vi "cRIO_EPTx_FPGA_MulInj_SCAN.vi"() -> ()   [LabVIEW 2023]
uses:
  C:/Program Files (x86)/National Instruments/LabVIEW 2023/vi.lib/Powertrain Controls/Device Drivers/Engine Position Tracking/EPTx/RevA/FPGA/Controls/EPTxDebug.ctl
  C:/Program Files (x86)/National Instruments/LabVIEW 2023/vi.lib/Powertrain Controls/Device Drivers/Engine Position Tracking/EPTx/RevA/FPGA/Controls/EPTxTooth.ctl
  <vilib>/Powertrain Controls/Device Drivers/Engine Position Tracking/EPTx/RevA/FPGA/Controls/EPTxSignals.ctl
  <vilib>/Powertrain Controls/Device Drivers/Engine Position Tracking/EPTx/RevA/FPGA/Controls/EPTxSupervisor.ctl
  <vilib>/Platform/TimedLoop/XDataNode/timing_clust.ctl
  <vilib>/Platform/TimedLoop/XDataNode/nitl_modes.ctl
  <vilib>/Platform/TimedLoop/XDataNode/wakeup.ctl
  <vilib>/Powertrain Controls/Device Drivers/Engine Position Tracking/EPTx/RevA/FPGA/Controls/EPTxAAPControl.ctl
  <vilib>/Powertrain Controls/Device Drivers/Engine Position Tracking/EPTx/RevA/FPGA/Controls/EPTxPatternConfig.ctl
  <vilib>/Powertrain Controls/Device Drivers/Engine Position Tracking/EPTx/RevA/FPGA/Controls/Patterns.ctl
  <vilib>/Powertrain Controls/Device Drivers/Engine Position Tracking/EPTx/RevA/FPGA/Controls/EPTxControl.ctl
  <vilib>/rvi/Emulation/niFpgaSctlEmulationGetInTimedLoop.vi
  <vilib>/rvi/Emulation/niFpgaEmulationReportErrorSimple.vi
  <vilib>/rvi/Emulation/niFpgaGetClockAttributes.vi
  <vilib>/rvi/Emulation/niFpgaCriticalErrorInLSC.vi
  <vilib>/rvi/eio/common/nirviEmuTemplateMethod_errors.vi
  <vilib>/Platform/TimedLoop/XDataNode/XDataNode.xnode
  <vilib>/eio/EIONode/EIONode.xnode
  <vilib>/Powertrain Controls/Device Drivers/Engine Position Tracking/EPTx/RevA/FPGA/Extras/Command Sequence - 12e.vi
  <vilib>/Platform/TimedLoop/XDataNode/XDNodeRunTimeDep.lvlib
  <vilib>/Powertrain Controls/Device Drivers/Engine Position Tracking/EPTx/RevA/FPGA/EPTx - RevA - FPGA.lvlib
panel:
  out "EPTxSupervisor_FPGA":T1
  out "EPTxSignals":T2
  out "EPTxTooth":T3
  out "EPTxDebug":T4
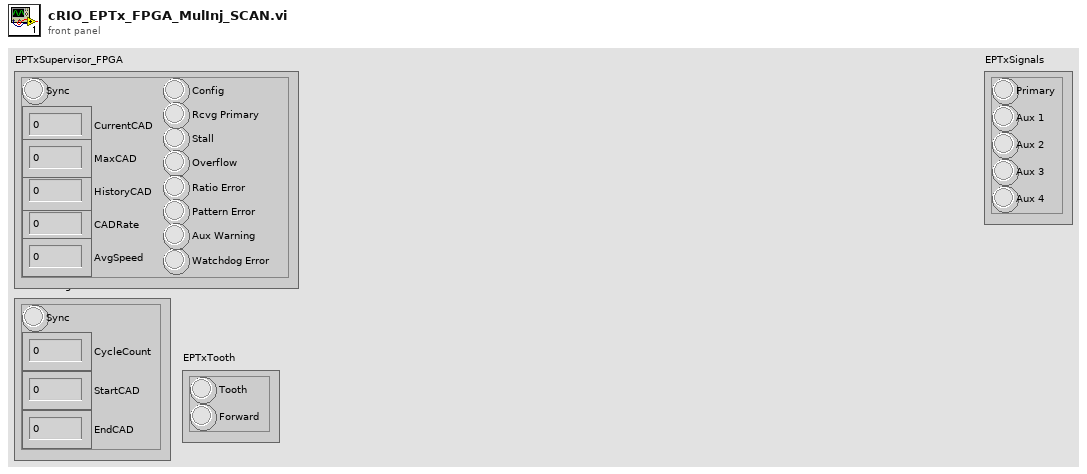
[diagram p1: front panel]
types:
  T1 = typedef "EPTx - RevA - FPGA.lvlib/EPTxSupervisor.ctl" = cluster{"Sync":bool, "CurrentCAD":fxp<+,18,11>, "MaxCAD":fxp<+,11,11>, "HistoryCAD":fxp<+,11,11>, "CADRate":fxp<+,22,8>, "AvgSpeed":fxp<+,17,15>, "Config":bool, "Rcvg Primary":bool, "Stall":bool, "Overflow":bool, "Ratio Error":bool, "Pattern Error":bool, "Aux Warning":bool, "Watchdog Error":bool}
  T2 = typedef "EPTx - RevA - FPGA.lvlib/EPTxSignals.ctl" = cluster{"Primary":bool, "Aux 1":bool, "Aux 2":bool, "Aux 3":bool, "Aux 4":bool}
  T3 = typedef "EPTxTooth.ctl" = cluster{"Tooth":bool, "Forward":bool}
  T4 = typedef "EPTx - RevA - FPGA.lvlib/EPTxDebug.ctl" = cluster{"Sync":bool, "CycleCount":fxp<+,8,8>, "StartCAD":fxp<+,18,11>, "EndCAD":fxp<+,18,11>}
  T5 = typedef "XDNodeRunTimeDep.lvlib/timing_clust.ctl" = cluster{"Expected End [f-1]":u64, "Actual End [f-1]":u64, "Finished Late? [f-1]":bool, "Expected End [i-1]":u64, "Actual End [i-1]":u64, "Finished Late? [i-1]":bool, "Expected Start [i]":u64, "Actual Start [i]":u64, "Expected Start [f]":u64, "Actual Start [f]":u64, "Source Name":string, "Structure Name":string, "Period":i64, "Deadline":i64, "Offset":i64, "Start":i64, "Priority":i32, "Timeout":i32, "Mode":T6, "Wakeup Reason":T7, "Error":errorcluster, "Source Type":string, "Secondary Source Type":string, "Global End Time":u64, "Global Start Time":u64, "Frame Duration":u64, "Iteration Duration":u64, "Assigned CPU":i32, "I/O Scan Engine Mode":u32}
  T6 = typedef "XDNodeRunTimeDep.lvlib/nitl_modes.ctl" = enum32{"No Change", "Process missed periods, maintain original phase", "Discard missed periods, maintain original phase", "Process missed periods, ignore original phase", "Discard missed periods, ignore original phase"}
  T7 = typedef "XDNodeRunTimeDep.lvlib/wakeup.ctl" = enum32{"Normal", "Aborted", "Asynchronous wakeup", "Timing source error", "Timed loop error", "Timeout"}
  T8 = typedef "EPTx - RevA - FPGA.lvlib/EPTxAAPControl.ctl" = cluster{"Enable":bool, "RisingCAD":fxp<+,18,11>, "FallingCAD":fxp<+,18,11>}
  T9 = typedef "EPTx - RevA - FPGA.lvlib/EPTxControl.ctl" = cluster{"Sync Enable":bool, "Clear Errors":bool, "Sim Enable":bool, "Sim Rate":fxp<+,24,6>, "Watchdog":bool}
  T10 = typedef "EPTx - RevA - FPGA.lvlib/Patterns.ctl" = cluster{"Primary":fxp<+,19,12>, "Primary State":bool, "Aux 1":fxp<+,19,12>, "Aux 1 State":bool, "Aux 2":fxp<+,19,12>, "Aux 2 State":bool, "Aux 3":fxp<+,19,12>, "Aux 3 State":bool, "Aux 4":fxp<+,19,12>, "Aux 4 State":bool}
  T11 = typedef "EPTx - RevA - FPGA.lvlib/EPTxPatternConfig.ctl" = cluster{"Address":fxp<+,14,14>, "Pattern":T10}
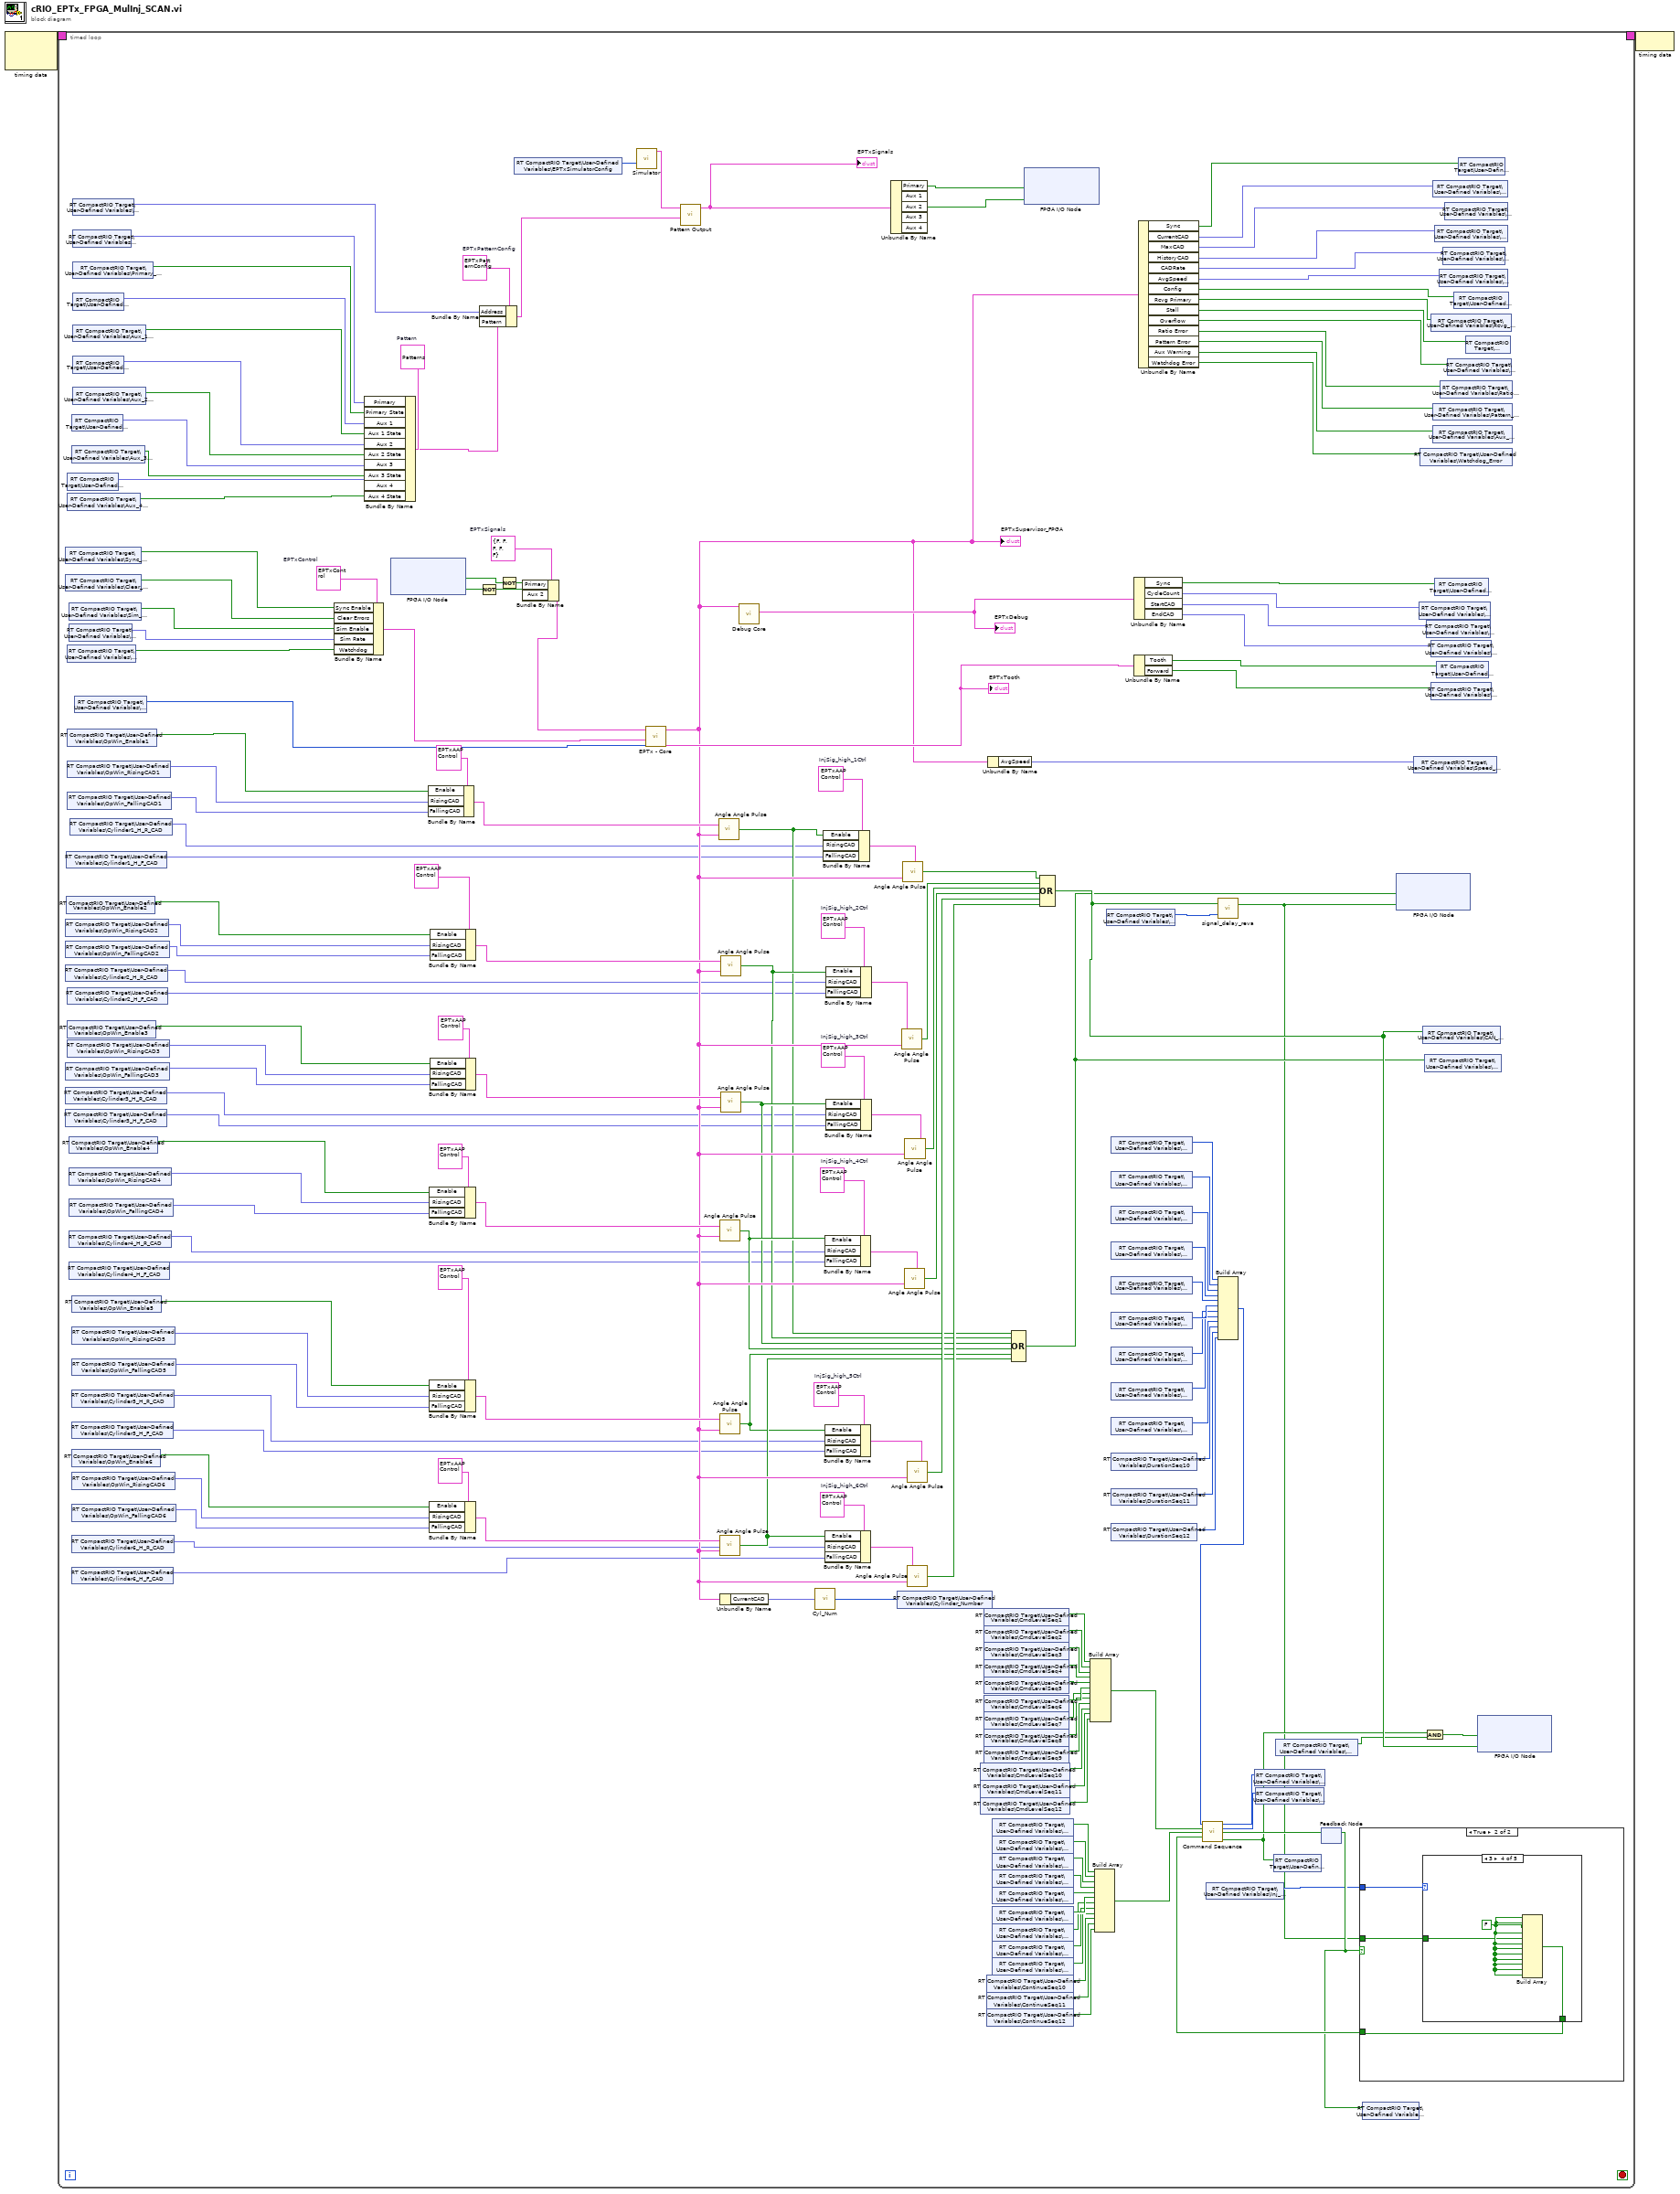
[diagram p0: block diagram]
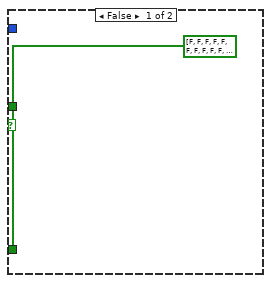
[diagram p2: hidden frame]
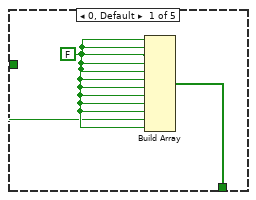
[diagram p3: hidden frame]
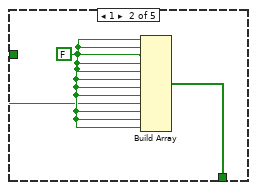
[diagram p4: hidden frame]
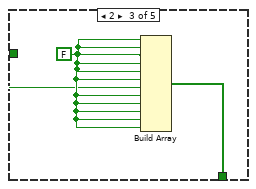
[diagram p5: hidden frame]
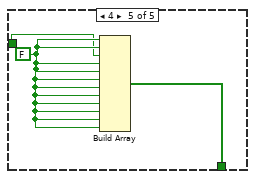
[diagram p6: hidden frame]
diagram:
  n1 = node-c288() -> (w2:T5)  [unwired: 2 in]
  n2 = timed-loop {
    timing: w2 -> [_]
    timing-out: [_] -> w1
    stop <- _ stop-if-true
    w139 = T2 {"Primary"=FALSE, "Aux 1"=FALSE, "Aux 2"=FALSE, "Aux 3"=FALSE, "Aux 4"=FALSE}  # EPTxSignals
    w145 = T8 {"Enable"=FALSE, "RisingCAD"=0.0, "FallingCAD"=0.0}  # InjSig_high_6Ctrl
    w150 = T8 {"Enable"=FALSE, "RisingCAD"=0.0, "FallingCAD"=0.0}  # InjSig_high_5Ctrl
    w153 = T8 {"Enable"=FALSE, "RisingCAD"=0.0, "FallingCAD"=0.0}  # InjSig_high_4Ctrl
    w160 = T8 {"Enable"=FALSE, "RisingCAD"=0.0, "FallingCAD"=0.0}  # InjSig_high_3Ctrl
    w164 = T8 {"Enable"=FALSE, "RisingCAD"=0.0, "FallingCAD"=0.0}  # InjSig_high_2Ctrl
    w168 = T9 {"Sync Enable"=FALSE, "Clear Errors"=FALSE, "Sim Enable"=FALSE, "Sim Rate"=0.0, "Watchdog"=FALSE}  # EPTxControl
    w173 = T10 {"Primary"=0.0, "Primary State"=FALSE, "Aux 1"=0.0, "Aux 1 State"=FALSE, "Aux 2"=0.0, "Aux 2 State"=FALSE, "Aux 3"=0.0, "Aux 3 State"=FALSE, "Aux 4"=0.0, "Aux 4 State"=FALSE}  # Pattern
    w174 = T11 {"Address"=0.0, "Pattern"={"Primary"=0.0, "Primary State"=FALSE, "Aux 1"=0.0, "Aux 1 State"=FALSE, "Aux 2"=0.0, "Aux 2 State"=FALSE, "Aux 3"=0.0, "Aux 3 State"=FALSE, "Aux 4"=0.0, "Aux 4 State"=FALSE}}  # EPTxPatternConfig
    w177 = T8 {"Enable"=FALSE, "RisingCAD"=0.0, "FallingCAD"=0.0}  # InjSig_high_1Ctrl
    n3 = shared-variable "RT CompactRIO Target\\User-Defined Variables\\OpWin_FallingCAD2"() -> (w103:fxp<+/-,32,16>)  [unwired: 1 in, 1 out]
    n4 = shared-variable "RT CompactRIO Target\\User-Defined Variables\\Cylinder3_H_R_CAD"() -> (w97:fxp<+/-,32,16>)  [unwired: 1 in, 1 out]
    n5 = shared-variable "RT CompactRIO Target\\User-Defined Variables\\Sync_Enable"() -> (w116:bool)  [unwired: 1 in, 1 out]
    n6 = shared-variable "RT CompactRIO Target\\User-Defined Variables\\Clear_Errors"() -> (w115:bool)  [unwired: 1 in, 1 out]
    n7 = shared-variable "RT CompactRIO Target\\User-Defined Variables\\OpWin_RisingCAD2"() -> (w104:fxp<+/-,32,16>)  [unwired: 1 in, 1 out]
    n8 = shared-variable "RT CompactRIO Target\\User-Defined Variables\\Cylinder2_H_R_CAD"() -> (w102:fxp<+/-,32,16>)  [unwired: 1 in, 1 out]
    n9 = shared-variable "RT CompactRIO Target\\User-Defined Variables\\OpWin_FallingCAD3"() -> (w98:fxp<+/-,32,16>)  [unwired: 1 in, 1 out]
    n10 = shared-variable "RT CompactRIO Target\\User-Defined Variables\\Cylinder3_H_F_CAD"() -> (w96:fxp<+/-,32,16>)  [unwired: 1 in, 1 out]
    n11 = shared-variable "RT CompactRIO Target\\User-Defined Variables\\Cylinder1_H_F_CAD"() -> (w106:fxp<+/-,32,16>)  [unwired: 1 in, 1 out]
    n12 = shared-variable "RT CompactRIO Target\\User-Defined Variables\\OpWin_Enable2"() -> (w105:bool)  [unwired: 1 in, 1 out]
    n13 = shared-variable "RT CompactRIO Target\\User-Defined Variables\\Aux_4"() -> (w119:fxp<+/-,32,16>)  [unwired: 1 in, 1 out]
    n14 = shared-variable "RT CompactRIO Target\\User-Defined Variables\\Aux_4_State"() -> (w118:bool)  [unwired: 1 in, 1 out]
    n15 = shared-variable "RT CompactRIO Target\\User-Defined Variables\\Watchdog"() -> (w112:bool)  [unwired: 1 in, 1 out]
    n16 = shared-variable "RT CompactRIO Target\\User-Defined Variables\\Cylinder2_H_F_CAD"() -> (w101:fxp<+/-,32,16>)  [unwired: 1 in, 1 out]
    n17 = shared-variable "RT CompactRIO Target\\User-Defined Variables\\OpWin_Enable3"() -> (w100:bool)  [unwired: 1 in, 1 out]
    n18 = shared-variable "RT CompactRIO Target\\User-Defined Variables\\OpWin_RisingCAD3"() -> (w99:fxp<+/-,32,16>)  [unwired: 1 in, 1 out]
    n19 = shared-variable "RT CompactRIO Target\\User-Defined Variables\\OpWin_Enable1"() -> (w110:bool)  [unwired: 1 in, 1 out]
    n20 = shared-variable "RT CompactRIO Target\\User-Defined Variables\\OpWin_RisingCAD1"() -> (w109:fxp<+/-,32,16>)  [unwired: 1 in, 1 out]
    n21 = shared-variable "RT CompactRIO Target\\User-Defined Variables\\OpWin_FallingCAD1"() -> (w108:fxp<+/-,32,16>)  [unwired: 1 in, 1 out]
    n22 = shared-variable "RT CompactRIO Target\\User-Defined Variables\\Sim_Enable"() -> (w114:bool)  [unwired: 1 in, 1 out]
    n23 = shared-variable "RT CompactRIO Target\\User-Defined Variables\\Sim_Rate"() -> (w113:fxp<+/-,16,7>)  [unwired: 1 in, 1 out]
    n24 = shared-variable "RT CompactRIO Target\\User-Defined Variables\\OpWin_Enable4"() -> (w95:bool)  [unwired: 1 in, 1 out]
    n25 = shared-variable "RT CompactRIO Target\\User-Defined Variables\\OpWin_RisingCAD4"() -> (w94:fxp<+/-,32,16>)  [unwired: 1 in, 1 out]
    n26 = shared-variable "RT CompactRIO Target\\User-Defined Variables\\OpWin_FallingCAD4"() -> (w93:fxp<+/-,32,16>)  [unwired: 1 in, 1 out]
    n27 = shared-variable "RT CompactRIO Target\\User-Defined Variables\\Cylinder4_H_R_CAD"() -> (w92:fxp<+/-,32,16>)  [unwired: 1 in, 1 out]
    n28 = shared-variable "RT CompactRIO Target\\User-Defined Variables\\Cylinder4_H_F_CAD"() -> (w91:fxp<+/-,32,16>)  [unwired: 1 in, 1 out]
    n29 = shared-variable "RT CompactRIO Target\\User-Defined Variables\\Cylinder1_H_R_CAD"() -> (w107:fxp<+/-,32,16>)  [unwired: 1 in, 1 out]
    n30 = shared-variable "RT CompactRIO Target\\User-Defined Variables\\Aux_3"() -> (w121:fxp<+/-,32,16>)  [unwired: 1 in, 1 out]
    n31 = shared-variable "RT CompactRIO Target\\User-Defined Variables\\Aux_3_State"() -> (w120:bool)  [unwired: 1 in, 1 out]
    n32 = shared-variable "RT CompactRIO Target\\User-Defined Variables\\OpWin_Enable6"() -> (w86:bool)  [unwired: 1 in, 1 out]
    n33 = shared-variable "RT CompactRIO Target\\User-Defined Variables\\OpWin_Enable5"() -> (w90:bool)  [unwired: 1 in, 1 out]
    n34 = shared-variable "RT CompactRIO Target\\User-Defined Variables\\OpWin_RisingCAD5"() -> (w6:fxp<+/-,32,16>)  [unwired: 1 in, 1 out]
    n35 = shared-variable "RT CompactRIO Target\\User-Defined Variables\\OpWin_FallingCAD5"() -> (w89:fxp<+/-,32,16>)  [unwired: 1 in, 1 out]
    n36 = shared-variable "RT CompactRIO Target\\User-Defined Variables\\Cylinder5_H_R_CAD"() -> (w88:fxp<+/-,32,16>)  [unwired: 1 in, 1 out]
    n37 = shared-variable "RT CompactRIO Target\\User-Defined Variables\\Cylinder5_H_F_CAD"() -> (w87:fxp<+/-,32,16>)  [unwired: 1 in, 1 out]
    n38 = shared-variable "RT CompactRIO Target\\User-Defined Variables\\OpWin_RisingCAD6"() -> (w85:fxp<+/-,32,16>)  [unwired: 1 in, 1 out]
    n39 = shared-variable "RT CompactRIO Target\\User-Defined Variables\\OpWin_FallingCAD6"() -> (w84:fxp<+/-,32,16>)  [unwired: 1 in, 1 out]
    n40 = shared-variable "RT CompactRIO Target\\User-Defined Variables\\Cylinder6_H_R_CAD"() -> (w83:fxp<+/-,32,16>)  [unwired: 1 in, 1 out]
    n41 = shared-variable "RT CompactRIO Target\\User-Defined Variables\\Cylinder6_H_F_CAD"() -> (w82:fxp<+/-,32,16>)  [unwired: 1 in, 1 out]
    n42 = shared-variable "RT CompactRIO Target\\User-Defined Variables\\Address"() -> (w128:fxp<+/-,32,16>)  [unwired: 1 in, 1 out]
    n43 = shared-variable "RT CompactRIO Target\\User-Defined Variables\\Primary"() -> (w127:fxp<+/-,32,16>)  [unwired: 1 in, 1 out]
    n44 = shared-variable "RT CompactRIO Target\\User-Defined Variables\\Primary_State"() -> (w126:bool)  [unwired: 1 in, 1 out]
    n45 = shared-variable "RT CompactRIO Target\\User-Defined Variables\\Aux_1"() -> (w125:fxp<+/-,32,16>)  [unwired: 1 in, 1 out]
    n46 = shared-variable "RT CompactRIO Target\\User-Defined Variables\\Aux_1_State"() -> (w124:bool)  [unwired: 1 in, 1 out]
    n47 = shared-variable "RT CompactRIO Target\\User-Defined Variables\\Aux_2"() -> (w123:fxp<+/-,32,16>)  [unwired: 1 in, 1 out]
    n48 = shared-variable "RT CompactRIO Target\\User-Defined Variables\\Aux_2_State"() -> (w122:bool)  [unwired: 1 in, 1 out]
    n49 = shared-variable "RT CompactRIO Target\\User-Defined Variables\\EPTxConfig"() -> (w111:u64)  [unwired: 1 in, 1 out]
    n50 = Bundle By Name(cluster=w168, "Sync Enable"=w116, "Clear Errors"=w115, "Sim Enable"=w114, "Sim Rate"=w113, "Watchdog"=w112) -> (w167:T9)
    n51 = Bundle By Name(cluster=w173, "Primary"=w127, "Primary State"=w126, "Aux 1"=w125, "Aux 1 State"=w124, "Aux 2"=w123, "Aux 2 State"=w122, "Aux 3"=w121, "Aux 3 State"=w120, "Aux 4"=w119, "Aux 4 State"=w118) -> (w172:T10)
    n52 = xnode "FPGA I/O Node"() -> ("Mod7/DIO0"=w31:bool, "Mod7/DIO1"=w29:bool)  [unwired: 2 in, 2 out]
    n53 = Bundle By Name(cluster=T8 {"Enable"=FALSE, "RisingCAD"=0.0, "FallingCAD"=0.0} ("AAPControl_1str"), "Enable"=w110, "RisingCAD"=w109, "FallingCAD"=w108) -> (w169:T8)
    n54 = Bundle By Name(cluster=T8 {"Enable"=FALSE, "RisingCAD"=0.0, "FallingCAD"=0.0} ("AAPControl_1str"), "Enable"=w95, "RisingCAD"=w94, "FallingCAD"=w93) -> (w155:T8)
    n55 = Bundle By Name(cluster=T8 {"Enable"=FALSE, "RisingCAD"=0.0, "FallingCAD"=0.0} ("AAPControl_1str"), "Enable"=w90, "RisingCAD"=w6, "FallingCAD"=w89) -> (w148:T8)
    n56 = Bundle By Name(cluster=T8 {"Enable"=FALSE, "RisingCAD"=0.0, "FallingCAD"=0.0} ("AAPControl_1str"), "Enable"=w86, "RisingCAD"=w85, "FallingCAD"=w84) -> (w147:T8)
    n57 = Bundle By Name(cluster=T8 {"Enable"=FALSE, "RisingCAD"=0.0, "FallingCAD"=0.0} ("AAPControl_1str"), "Enable"=w105, "RisingCAD"=w104, "FallingCAD"=w103) -> (w166:T8)
    n58 = Bundle By Name(cluster=T8 {"Enable"=FALSE, "RisingCAD"=0.0, "FallingCAD"=0.0} ("AAPControl_1str"), "Enable"=w100, "RisingCAD"=w99, "FallingCAD"=w98) -> (w158:T8)
    n59 = Bundle By Name(cluster=w174, "Address"=w128, "Pattern"=w172) -> (w171:T11)
    n60 = Not(x=w29) -> (.not. x?=w28:bool)
    n61 = Not(x=w31) -> (.not. x?=w30:bool)
    n62 = shared-variable "RT CompactRIO Target\\User-Defined Variables\\EPTxSimulatorConfig"() -> (w117:u32)  [unwired: 1 in, 1 out]
    n63 = Bundle By Name(cluster=w139, "Primary"=w30, "Aux 2"=w28) -> (w138:T2)
    n64 = call <vilib>:"Simulator.vi"("EPTxSimulatorConfig"=w117) -> ("EPTxSupervisor"=w180:T1)  [unwired: 10 in]
    n65 = call <vilib>:"EPTx - Core.vi"("EPTxConfig"=w111, "EPTxControl"=w167, "EPTxSignals"=w138) -> ("EPTxTooth"=w175:T3, "EPTxSupervisor"=w140:T1)  [unwired: 7 in]
    "EPTxSupervisor_FPGA" <- w140
    "EPTxTooth" <- w175
    n66 = call <vilib>:"Pattern Output.vi"("EPTxPatternConfig"=w171, "EPTxSupervisor"=w180) -> ("PatternOutput"=w179:T2)  [unwired: 9 in]
    "EPTxSignals" <- w179
    n67 = call <vilib>:"Angle Angle Pulse.vi"("EPTxSupervisor"=w140, "AAPControl"=w169) -> ("AAP"=w132:bool)
    n68 = call <vilib>:"Angle Angle Pulse.vi"("EPTxSupervisor"=w140, "AAPControl"=w155) -> ("AAP"=w135:bool)
    n69 = call <vilib>:"Angle Angle Pulse.vi"("EPTxSupervisor"=w140, "AAPControl"=w148) -> ("AAP"=w136:bool)
    n70 = call <vilib>:"Angle Angle Pulse.vi"("EPTxSupervisor"=w140, "AAPControl"=w147) -> ("AAP"=w137:bool)
    n71 = Unbundle By Name(w140) -> ("CurrentCAD"=w27:fxp<+,18,11>)
    n72 = call <vilib>:"Angle Angle Pulse.vi"("EPTxSupervisor"=w140, "AAPControl"=w166) -> ("AAP"=w133:bool)
    n73 = call <vilib>:"Angle Angle Pulse.vi"("EPTxSupervisor"=w140, "AAPControl"=w158) -> ("AAP"=w134:bool)
    n74 = call <vilib>:"Debug Core.vi"("EPTxSupervisor"=w140) -> ("EPTxDebug"=w176:T4)  [unwired: 10 in]
    "EPTxDebug" <- w176
    n75 = call "Cyl_Num.vi"("CurrentCAD"=w27) -> ("Cylinder_Num"=w26:u8)
    n76 = Bundle By Name(cluster=w177, "Enable"=w132, "RisingCAD"=w107, "FallingCAD"=w106) -> (w178:T8)
    n77 = Bundle By Name(cluster=w153, "Enable"=w135, "RisingCAD"=w92, "FallingCAD"=w91) -> (w152:T8)
    n78 = Bundle By Name(cluster=w150, "Enable"=w136, "RisingCAD"=w88, "FallingCAD"=w87) -> (w151:T8)
    n79 = Bundle By Name(cluster=w145, "Enable"=w137, "RisingCAD"=w83, "FallingCAD"=w82) -> (w144:T8)
    n80 = Bundle By Name(cluster=w164, "Enable"=w133, "RisingCAD"=w102, "FallingCAD"=w101) -> (w163:T8)
    n81 = Bundle By Name(cluster=w160, "Enable"=w134, "RisingCAD"=w97, "FallingCAD"=w96) -> (w161:T8)
    n82 = Unbundle By Name(w179) -> ("Primary"=w33:bool, "Aux 2"=w32:bool)  [unwired: 3 out]
    n83 = shared-variable "RT CompactRIO Target\\User-Defined Variables\\Cylinder_Number"(w26) -> ()  [unwired: 1 in, 1 out]
    n84 = call <vilib>:"Angle Angle Pulse.vi"("EPTxSupervisor"=w140, "AAPControl"=w163) -> ("AAP"=w157:bool)
    n85 = call <vilib>:"Angle Angle Pulse.vi"("EPTxSupervisor"=w140, "AAPControl"=w178) -> ("AAP"=w162:bool)
    n86 = call <vilib>:"Angle Angle Pulse.vi"("EPTxSupervisor"=w140, "AAPControl"=w152) -> ("AAP"=w143:bool)
    n87 = call <vilib>:"Angle Angle Pulse.vi"("EPTxSupervisor"=w140, "AAPControl"=w161) -> ("AAP"=w156:bool)
    n88 = call <vilib>:"Angle Angle Pulse.vi"("EPTxSupervisor"=w140, "AAPControl"=w151) -> ("AAP"=w142:bool)
    n89 = call <vilib>:"Angle Angle Pulse.vi"("EPTxSupervisor"=w140, "AAPControl"=w144) -> ("AAP"=w141:bool)
    n90 = shared-variable "RT CompactRIO Target\\User-Defined Variables\\CmdLevelSeq10"() -> (w59:bool)  [unwired: 1 in, 1 out]
    n91 = shared-variable "RT CompactRIO Target\\User-Defined Variables\\CmdLevelSeq11"() -> (w58:bool)  [unwired: 1 in, 1 out]
    n92 = shared-variable "RT CompactRIO Target\\User-Defined Variables\\CmdLevelSeq12"() -> (w57:bool)  [unwired: 1 in, 1 out]
    n93 = shared-variable "RT CompactRIO Target\\User-Defined Variables\\CmdLevelSeq1"() -> (w68:bool)  [unwired: 1 in, 1 out]
    n94 = shared-variable "RT CompactRIO Target\\User-Defined Variables\\CmdLevelSeq2"() -> (w67:bool)  [unwired: 1 in, 1 out]
    n95 = shared-variable "RT CompactRIO Target\\User-Defined Variables\\CmdLevelSeq3"() -> (w66:bool)  [unwired: 1 in, 1 out]
    n96 = shared-variable "RT CompactRIO Target\\User-Defined Variables\\CmdLevelSeq4"() -> (w65:bool)  [unwired: 1 in, 1 out]
    n97 = shared-variable "RT CompactRIO Target\\User-Defined Variables\\CmdLevelSeq5"() -> (w64:bool)  [unwired: 1 in, 1 out]
    n98 = shared-variable "RT CompactRIO Target\\User-Defined Variables\\CmdLevelSeq6"() -> (w63:bool)  [unwired: 1 in, 1 out]
    n99 = shared-variable "RT CompactRIO Target\\User-Defined Variables\\CmdLevelSeq7"() -> (w62:bool)  [unwired: 1 in, 1 out]
    n100 = shared-variable "RT CompactRIO Target\\User-Defined Variables\\CmdLevelSeq8"() -> (w61:bool)  [unwired: 1 in, 1 out]
    n101 = shared-variable "RT CompactRIO Target\\User-Defined Variables\\CmdLevelSeq9"() -> (w60:bool)  [unwired: 1 in, 1 out]
    n102 = shared-variable "RT CompactRIO Target\\User-Defined Variables\\ContinueSeq10"() -> (w12:bool)  [unwired: 1 in, 1 out]
    n103 = shared-variable "RT CompactRIO Target\\User-Defined Variables\\ContinueSeq11"() -> (w11:bool)  [unwired: 1 in, 1 out]
    n104 = shared-variable "RT CompactRIO Target\\User-Defined Variables\\ContinueSeq12"() -> (w10:bool)  [unwired: 1 in, 1 out]
    n105 = Unbundle By Name(w140) -> ("AvgSpeed"=w37:fxp<+,17,15>)
    n106 = shared-variable "RT CompactRIO Target\\User-Defined Variables\\ContinueSeq1"() -> (w21:bool)  [unwired: 1 in, 1 out]
    n107 = shared-variable "RT CompactRIO Target\\User-Defined Variables\\ContinueSeq2"() -> (w20:bool)  [unwired: 1 in, 1 out]
    n108 = shared-variable "RT CompactRIO Target\\User-Defined Variables\\ContinueSeq3"() -> (w19:bool)  [unwired: 1 in, 1 out]
    n109 = shared-variable "RT CompactRIO Target\\User-Defined Variables\\ContinueSeq4"() -> (w18:bool)  [unwired: 1 in, 1 out]
    n110 = shared-variable "RT CompactRIO Target\\User-Defined Variables\\ContinueSeq5"() -> (w17:bool)  [unwired: 1 in, 1 out]
    n111 = shared-variable "RT CompactRIO Target\\User-Defined Variables\\ContinueSeq6"() -> (w16:bool)  [unwired: 1 in, 1 out]
    n112 = shared-variable "RT CompactRIO Target\\User-Defined Variables\\ContinueSeq7"() -> (w15:bool)  [unwired: 1 in, 1 out]
    n113 = shared-variable "RT CompactRIO Target\\User-Defined Variables\\ContinueSeq8"() -> (w14:bool)  [unwired: 1 in, 1 out]
    n114 = shared-variable "RT CompactRIO Target\\User-Defined Variables\\ContinueSeq9"() -> (w13:bool)  [unwired: 1 in, 1 out]
    n115 = Compound Arithmetic op=OR ("复合运算")(w132, w133, w134, w135, w136, w137) -> (w4:bool)
    n116 = xnode "FPGA I/O Node"("Mod6/DIO0"=w33, "Mod6/DIO1"=w32) -> ()  [unwired: 2 in, 2 out]
    n117 = Compound Arithmetic op=OR ("复合运算")(w162, w157, w156, w143, w142, w141) -> (w25:bool)
    n118 = Build Array(w68, w67, w66, w65, w64, w63, w62, w61, w60, w59, w58, w57) -> (w130:bool[])
    n119 = Build Array(w21, w20, w19, w18, w17, w16, w15, w14, w13, w12, w11, w10) -> (w129:bool[])
    n120 = shared-variable "RT CompactRIO Target\\User-Defined Variables\\Delay[tick]"() -> (w81:u32)  [unwired: 1 in, 1 out]
    n121 = shared-variable "RT CompactRIO Target\\User-Defined Variables\\DurationSeq1"() -> (w80:u32)  [unwired: 1 in, 1 out]
    n122 = shared-variable "RT CompactRIO Target\\User-Defined Variables\\DurationSeq2"() -> (w79:u32)  [unwired: 1 in, 1 out]
    n123 = shared-variable "RT CompactRIO Target\\User-Defined Variables\\DurationSeq3"() -> (w78:u32)  [unwired: 1 in, 1 out]
    n124 = shared-variable "RT CompactRIO Target\\User-Defined Variables\\DurationSeq4"() -> (w77:u32)  [unwired: 1 in, 1 out]
    n125 = shared-variable "RT CompactRIO Target\\User-Defined Variables\\DurationSeq5"() -> (w76:u32)  [unwired: 1 in, 1 out]
    n126 = shared-variable "RT CompactRIO Target\\User-Defined Variables\\DurationSeq6"() -> (w75:u32)  [unwired: 1 in, 1 out]
    n127 = shared-variable "RT CompactRIO Target\\User-Defined Variables\\DurationSeq7"() -> (w74:u32)  [unwired: 1 in, 1 out]
    n128 = shared-variable "RT CompactRIO Target\\User-Defined Variables\\DurationSeq8"() -> (w73:u32)  [unwired: 1 in, 1 out]
    n129 = shared-variable "RT CompactRIO Target\\User-Defined Variables\\DurationSeq9"() -> (w72:u32)  [unwired: 1 in, 1 out]
    n130 = shared-variable "RT CompactRIO Target\\User-Defined Variables\\DurationSeq10"() -> (w71:u32)  [unwired: 1 in, 1 out]
    n131 = shared-variable "RT CompactRIO Target\\User-Defined Variables\\DurationSeq11"() -> (w70:u32)  [unwired: 1 in, 1 out]
    n132 = shared-variable "RT CompactRIO Target\\User-Defined Variables\\DurationSeq12"() -> (w69:u32)  [unwired: 1 in, 1 out]
    n133 = Unbundle By Name(w176) -> ("Sync"=w34:bool, "CycleCount"=w42:fxp<+,8,8>, "StartCAD"=w41:fxp<+,18,11>, "EndCAD"=w40:fxp<+,18,11>)
    n134 = Unbundle By Name(w175) -> ("Tooth"=w39:bool, "Forward"=w38:bool)
    n135 = Unbundle By Name(w140) -> ("Sync"=w56:bool, "CurrentCAD"=w55:fxp<+,18,11>, "MaxCAD"=w54:fxp<+,11,11>, "HistoryCAD"=w53:fxp<+,11,11>, "CADRate"=w52:fxp<+,22,8>, "AvgSpeed"=w51:fxp<+,17,15>, "Config"=w50:bool, "Rcvg Primary"=w49:bool, "Stall"=w48:bool, "Overflow"=w47:bool, "Ratio Error"=w46:bool, "Pattern Error"=w45:bool, "Aux Warning"=w44:bool, "Watchdog Error"=w43:bool)
    n136 = shared-variable "RT CompactRIO Target\\User-Defined Variables\\Inj_DrvMode"() -> (w7:u32)  [unwired: 1 in, 1 out]
    n137 = call <vilib>:"signal_delay_reva.vi"("Delay"=w81, "InpSig"=w25) -> ("OutSig"=w3:bool)
    n138 = Build Array(w80, w79, w78, w77, w76, w75, w74, w73, w72, w71, w70, w69) -> (w131:u32[])
    n139 = shared-variable "RT CompactRIO Target\\User-Defined Variables\\GlobalTrigger"() -> (w23:bool)  [unwired: 1 in, 1 out]
    n140 = feedback #1() -> (w8:bool)  [unwired: 1 in]
    n141 = case shown="True" w8 {
      tunnel: w3 -> [_ w184]
      tunnel: [bool[] [FALSE, FALSE, FALSE, FALSE, FALSE, FALSE, FALSE, FALSE, FALSE, FALSE, FALSE, FALSE] w183] -> w22
      tunnel: w7 -> [_ w182]
      frame False {
      }
      frame True {
        n142 = case shown="3" w182 {
          tunnel: w184 -> [w186 w189 w192 w195 w198]
          tunnel: [w185 w188 w191 w194 w197] -> w183
          frame 0, Default {
            w187 = FALSE
            n143 = Build Array(w187, w187, w187, w187, w187, w187, w187, w187, w187, w187, w186, w187) -> (w185:bool[])
          }
          frame 1 {
            w190 = FALSE
            n144 = Build Array(w190, w190, w190, w190, w190, w190, w190, w190, w189, w190, w190, w190) -> (w188:bool[])
          }
          frame 2 {
            w193 = FALSE
            n145 = Build Array(w193, w193, w193, w193, w193, w193, w192, w193, w193, w193, w193, w193) -> (w191:bool[])
          }
          frame 3 {
            w196 = FALSE
            n146 = Build Array(w196, w196, w196, w196, w195, w196, w196, w196, w196, w196, w196, w196) -> (w194:bool[])
          }
          frame 4 {
            w199 = FALSE
            n147 = Build Array(w199, w199, w198, w199, w199, w199, w199, w199, w199, w199, w199, w199) -> (w197:bool[])
          }
        }
      }
    }
    n148 = call-poly <vilib>:"Command Sequence.vi"("DurationSeq"=w131, "CmdLevelSeq"=w130, "ContinueSeq"=w129, "ElementTriggers"=w22) -> ("SeqPointer"=w35:u8, "CmdTimer"=w36:u32, "Paused"=w9:bool, "Cmd"=w5:bool)  [unwired: 8 in]
    n149 = shared-variable "RT CompactRIO Target\\User-Defined Variables\\SeqPointer"(w35) -> ()  [unwired: 1 in, 1 out]
    n150 = shared-variable "RT CompactRIO Target\\User-Defined Variables\\CmdTimer"(w36) -> ()  [unwired: 1 in, 1 out]
    n151 = shared-variable "RT CompactRIO Target\\User-Defined Variables\\Cmd"(w5) -> ()  [unwired: 1 in, 1 out]
    n152 = feedback-in #1(w9) -> ()
    n153 = shared-variable "RT CompactRIO Target\\User-Defined Variables\\Paused"(w8) -> ()  [unwired: 1 in, 1 out]
    n154 = xnode "FPGA I/O Node"("Mod6/DIO2"=w4, "Mod6/DIO5"=w3) -> ()  [unwired: 2 in, 2 out]
    n155 = shared-variable "RT CompactRIO Target\\User-Defined Variables\\Speed_Output"(w37) -> ()  [unwired: 1 in, 1 out]
    n156 = shared-variable "RT CompactRIO Target\\User-Defined Variables\\CycleCount"(w42) -> ()  [unwired: 1 in, 1 out]
    n157 = shared-variable "RT CompactRIO Target\\User-Defined Variables\\Watchdog_Error"(w43) -> ()  [unwired: 1 in, 1 out]
    n158 = shared-variable "RT CompactRIO Target\\User-Defined Variables\\CAN_Trigger"(w25) -> ()  [unwired: 1 in, 1 out]
    n159 = shared-variable "RT CompactRIO Target\\User-Defined Variables\\OpenWinSig"(w4) -> ()  [unwired: 1 in, 1 out]
    n160 = And(x=w5, y=w23) -> (x .and. y?=w24:bool)
    n161 = shared-variable "RT CompactRIO Target\\User-Defined Variables\\StartCAD"(w41) -> ()  [unwired: 1 in, 1 out]
    n162 = shared-variable "RT CompactRIO Target\\User-Defined Variables\\Forward"(w38) -> ()  [unwired: 1 in, 1 out]
    n163 = shared-variable "RT CompactRIO Target\\User-Defined Variables\\Rcvg_Primary"(w49) -> ()  [unwired: 1 in, 1 out]
    n164 = shared-variable "RT CompactRIO Target\\User-Defined Variables\\EndCAD"(w40) -> ()  [unwired: 1 in, 1 out]
    n165 = shared-variable "RT CompactRIO Target\\User-Defined Variables\\Pattern_Error"(w45) -> ()  [unwired: 1 in, 1 out]
    n166 = shared-variable "RT CompactRIO Target\\User-Defined Variables\\CurrentCAD"(w55) -> ()  [unwired: 1 in, 1 out]
    n167 = shared-variable "RT CompactRIO Target\\User-Defined Variables\\Aux_Warning"(w44) -> ()  [unwired: 1 in, 1 out]
    n168 = shared-variable "RT CompactRIO Target\\User-Defined Variables\\HistoryCAD"(w53) -> ()  [unwired: 1 in, 1 out]
    n169 = shared-variable "RT CompactRIO Target\\User-Defined Variables\\Sync_2"(w34) -> ()  [unwired: 1 in, 1 out]
    n170 = shared-variable "RT CompactRIO Target\\User-Defined Variables\\Tooth"(w39) -> ()  [unwired: 1 in, 1 out]
    n171 = shared-variable "RT CompactRIO Target\\User-Defined Variables\\AvgSpeed"(w51) -> ()  [unwired: 1 in, 1 out]
    n172 = shared-variable "RT CompactRIO Target\\User-Defined Variables\\Ratio_Error"(w46) -> ()  [unwired: 1 in, 1 out]
    n173 = shared-variable "RT CompactRIO Target\\User-Defined Variables\\CADRate"(w52) -> ()  [unwired: 1 in, 1 out]
    n174 = shared-variable "RT CompactRIO Target\\User-Defined Variables\\MaxCAD"(w54) -> ()  [unwired: 1 in, 1 out]
    n175 = shared-variable "RT CompactRIO Target\\User-Defined Variables\\Overflow"(w47) -> ()  [unwired: 1 in, 1 out]
    n176 = shared-variable "RT CompactRIO Target\\User-Defined Variables\\Config"(w50) -> ()  [unwired: 1 in, 1 out]
    n177 = shared-variable "RT CompactRIO Target\\User-Defined Variables\\Sync"(w56) -> ()  [unwired: 1 in, 1 out]
    n178 = shared-variable "RT CompactRIO Target\\User-Defined Variables\\Stall"(w48) -> ()  [unwired: 1 in, 1 out]
    n179 = xnode "FPGA I/O Node"("Mod6/DIO3"=w24, "Mod6/DIO4"=w25) -> ()  [unwired: 2 in, 2 out]
  }
  n180 = node-c288(w1) -> ()
